vi "Experiment 7.VI"() -> ()   [LabVIEW 2017]
uses:
  <vilib>/DAQmx/write.llb/DAQmx Write (Analog DBL 1Chan 1Samp).vi
  <vilib>/DAQmx/write.llb/DAQmx Write (Digital 1D Bool NChan 1Samp 1Line).vi
  <vilib>/DAQmx/read.llb/DAQmx Read (Digital 1D Bool NChan 1Samp 1Line).vi
  <vilib>/DAQmx/read.llb/DAQmx Read (Analog 2D DBL NChan NSamp).vi
  <vilib>/DAQmx/create/channels.llb/DAQmx Create Channel (DI-Digital Input).vi
  <vilib>/DAQmx/create/channels.llb/DAQmx Create Channel (AI-Voltage-Basic).vi
  <vilib>/DAQmx/configure/timing.llb/DAQmx Timing (Sample Clock).vi
  <vilib>/DAQmx/create/channels.llb/DAQmx Create Channel (AO-Voltage-Basic).vi
  <vilib>/DAQmx/create/channels.llb/DAQmx Create Channel (DO-Digital Output).vi
  <vilib>/DAQmx/miscellaneous.llb/DAQmx Fill In Error Info.vi
panel:
  in  "Analogue Output":dbl(slide) scale=0.0..10.0
  out "Analogue Loopback":dbl[](graph)
  in  "Red LED":bool
  in  "Green LED":bool
  out "Button":bool
  out "Switch":bool
  in  "stop":bool
  out "Potentionmeter":dbl[](graph)
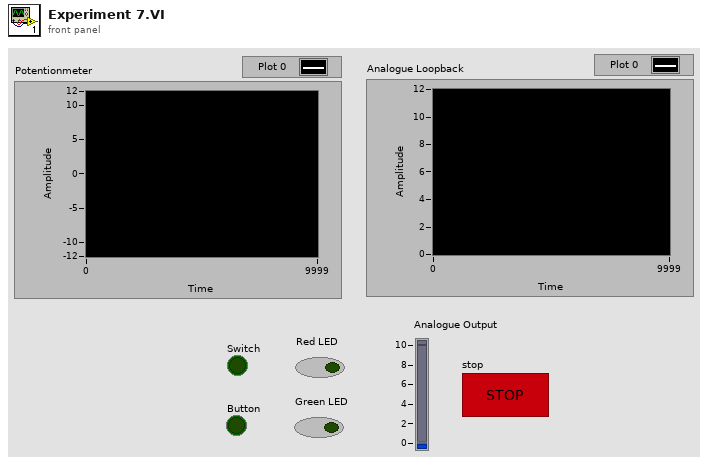
[diagram p1: front panel]
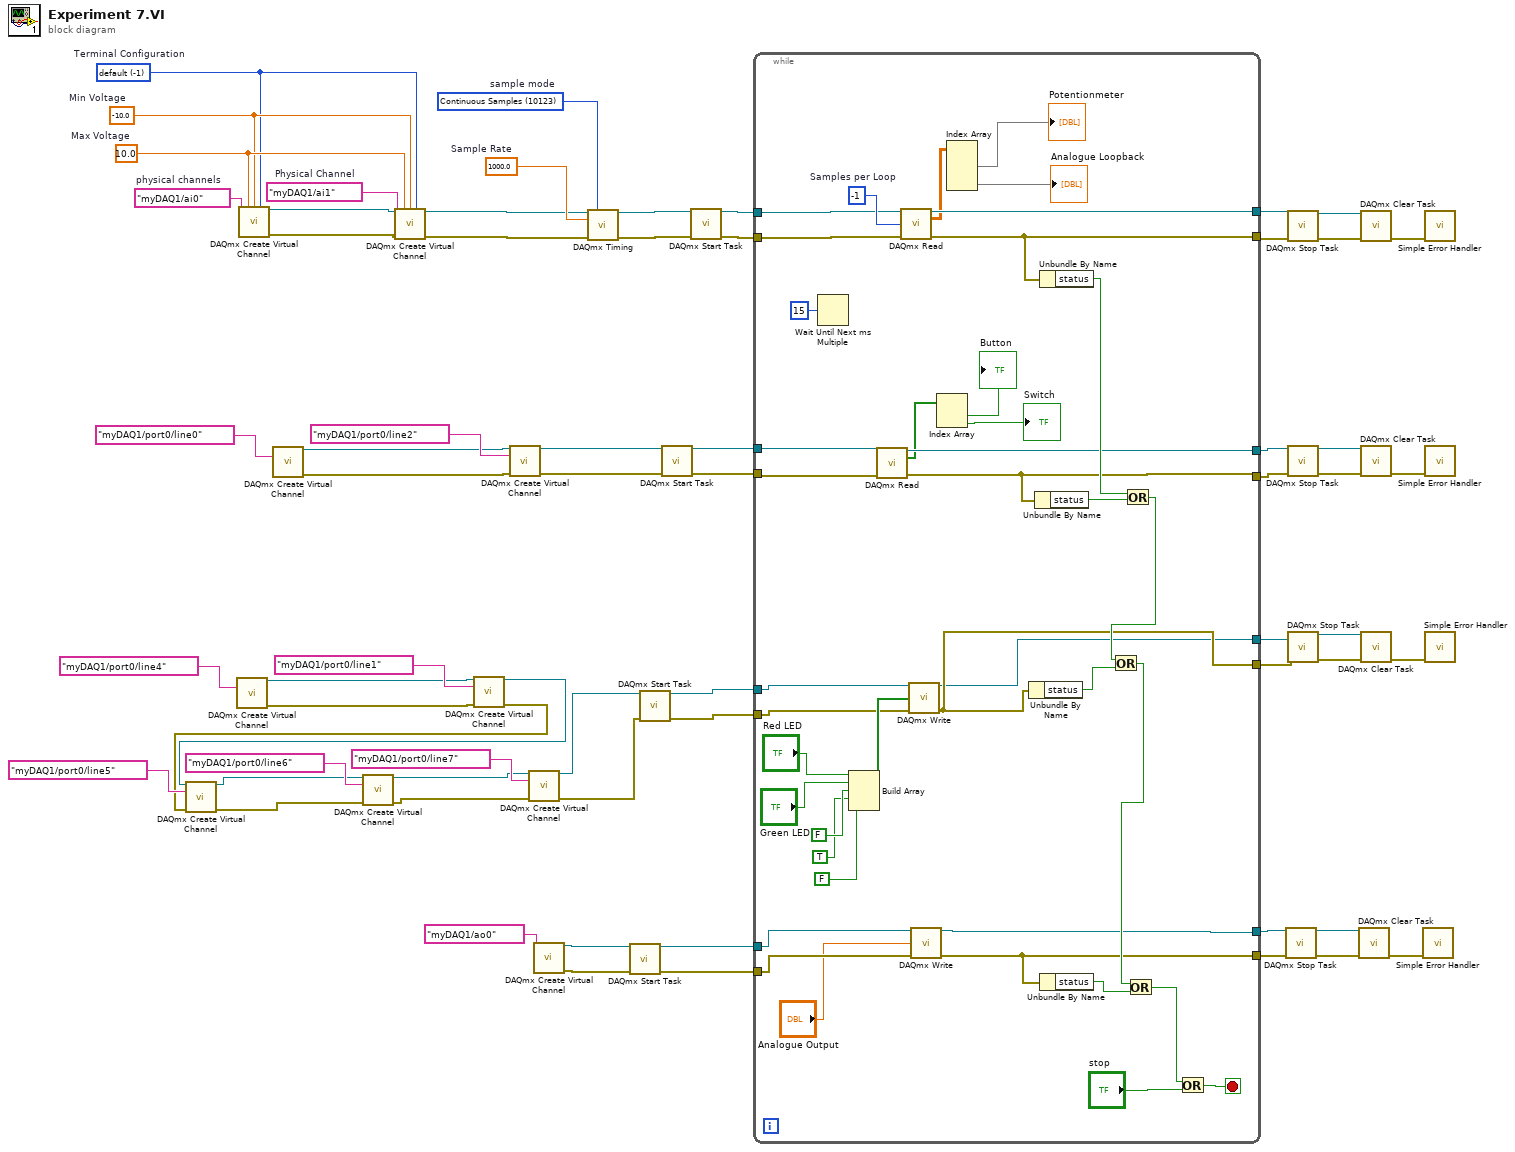
[diagram p0: block diagram]
diagram:
  w29 = tag "myDAQ1/ai0"  # physical channels
  w63 = 10123 items=["Finite Samples"=10178, "Continuous Samples"=10123, "Hardware Timed Single Point"=12522]  # sample mode
  w64 = 1000.0  # Sample Rate
  w26 = -1 items=["default"=-1, "RSE"=10083, "NRSE"=10078, "Differential"=10106, "Pseudodifferential"=12529]  # Terminal Configuration
  w27 = -10.0  # Min Voltage
  w28 = 10.0  # Max Voltage
  w65 = tag "myDAQ1/ai1"  # Physical Channel
  n1 = call-poly <vilib>:"DAQmx Create Virtual Channel.vi"("lines"=tag "myDAQ1/port0/line4") -> ("task out"=w16:refnum<k21>, "error out"=w15:errorcluster)  [unwired: 13 in]
  n2 = call-poly <vilib>:"DAQmx Create Virtual Channel.vi"("maximum value"=w28, "minimum value"=w27, "input terminal configuration"=w26, "physical channels"=w29) -> ("task out"=w30:refnum<k21>, "error out"=w31:errorcluster)  [unwired: 10 in]
  n3 = call-poly <vilib>:"DAQmx Create Virtual Channel.vi"("lines"=tag "myDAQ1/port0/line0") -> ("task out"=w41:refnum<k21>, "error out"=w40:errorcluster)  [unwired: 13 in]
  n4 = call-poly <vilib>:"DAQmx Create Virtual Channel.vi"("task in"=w30, "maximum value"=w28, "minimum value"=w27, "input terminal configuration"=w26, "physical channels"=w65, "error in"=w31) -> ("task out"=w61:refnum<k21>, "error out"=w62:errorcluster)  [unwired: 8 in]
  n5 = call-poly <vilib>:"DAQmx Create Virtual Channel.vi"("task in"=w16, "lines"=tag "myDAQ1/port0/line1", "error in"=w15) -> ("task out"=w10:refnum<k21>, "error out"=w5:errorcluster)  [unwired: 11 in]
  n6 = call-poly <vilib>:"DAQmx Create Virtual Channel.vi"("task in"=w10, "lines"=tag "myDAQ1/port0/line5", "error in"=w5) -> ("task out"=w9:refnum<k21>, "error out"=w6:errorcluster)  [unwired: 11 in]
  n7 = call-poly <vilib>:"DAQmx Create Virtual Channel.vi"("task in"=w9, "lines"=tag "myDAQ1/port0/line6", "error in"=w6) -> ("task out"=w8:refnum<k21>, "error out"=w7:errorcluster)  [unwired: 11 in]
  n8 = call-poly <vilib>:"DAQmx Create Virtual Channel.vi"("task in"=w41, "lines"=tag "myDAQ1/port0/line2", "error in"=w40) -> ("task out"=w50:refnum<k21>, "error out"=w49:errorcluster)  [unwired: 11 in]
  n9 = call-poly <vilib>:"DAQmx Create Virtual Channel.vi"("task in"=w8, "lines"=tag "myDAQ1/port0/line7", "error in"=w7) -> ("task out"=w4:refnum<k21>, "error out"=w3:errorcluster)  [unwired: 11 in]
  n10 = call-poly <vilib>:"DAQmx Create Virtual Channel.vi"("physical channels"=tag "myDAQ1/ao0") -> ("task out"=w22:refnum<k21>, "error out"=w21:errorcluster)  [unwired: 13 in]
  n11 = call-poly <vilib>:"DAQmx Timing.vi"("task/channels in"=w61, "sample mode"=w63, "rate"=w64, "error in"=w62) -> ("task out"=w60:refnum<k21>, "error out"=w59:errorcluster)  [unwired: 10 in]
  n12 = call <vilib>:"DAQmx Start Task.vi"("task/channels in"=w22, "error in"=w21) -> ("task out"=w19:refnum<k21>, "error out"=w18:errorcluster)  [unwired: 12 in]
  n13 = call <vilib>:"DAQmx Start Task.vi"("task/channels in"=w4, "error in"=w3) -> ("task out"=w33:refnum<k21>, "error out"=w32:errorcluster)  [unwired: 12 in]
  n14 = call <vilib>:"DAQmx Start Task.vi"("task/channels in"=w50, "error in"=w49) -> ("task out"=w48:refnum<k21>, "error out"=w47:errorcluster)  [unwired: 12 in]
  n15 = call <vilib>:"DAQmx Start Task.vi"("task/channels in"=w60, "error in"=w59) -> ("task out"=w58:refnum<k21>, "error out"=w57:errorcluster)  [unwired: 12 in]
  n16 = while {
    tunnel: w58 -> [w102]
    tunnel: w57 -> [w103]
    tunnel: [w99] -> w54
    tunnel: [w98] -> w53
    tunnel: w48 -> [w96]
    tunnel: w47 -> [w95]
    tunnel: [w94] -> w43
    tunnel: [w92] -> w42
    tunnel: [w86] -> w37
    tunnel: [w85] -> w38
    tunnel: w33 -> [w82]
    tunnel: w32 -> [w83]
    tunnel: w19 -> [w69]
    tunnel: w18 -> [w68]
    tunnel: [w70] -> w1
    tunnel: [w67] -> w2
    stop <- w101 stop-if-true
    w104 = -1  # Samples per Loop
    n17 = Wait Until Next ms Multiple(millisecond multiple=u32 15) -> ()  [unwired: 1 out]
    n18 = Build Array("Red LED", "Green LED", FALSE, TRUE, FALSE) -> (w84:bool[])
    n19 = call-poly <vilib>:"DAQmx Read.vi"("task/channels in"=w96, "error in"=w95) -> ("task out"=w92:refnum<k21>, "data"=w91:bool[], "error out"=w94:errorcluster)  [unwired: 11 in]
    n20 = call-poly <vilib>:"DAQmx Read.vi"("task/channels in"=w102, "number of samples per channel"=w104, "error in"=w103) -> ("task out"=w98:refnum<k21>, "data"=w78:dbl[][], "error out"=w99:errorcluster)  [unwired: 10 in]
    n21 = call-poly <vilib>:"DAQmx Write.vi"("task/channels in"=w82, "data"=w84, "error in"=w83) -> ("task out"=w85:refnum<k21>, "error out"=w86:errorcluster)  [unwired: 10 in, 1 out]
    n22 = call-poly <vilib>:"DAQmx Write.vi"("task/channels in"=w69, "data"="Analogue Output", "error in"=w68) -> ("task out"=w67:refnum<k21>, "error out"=w70:errorcluster)  [unwired: 10 in, 1 out]
    n23 = Index Array(array=w91) -> (element #1=→"Button":bool, element #2=→"Switch":bool)  [unwired: 2 in]
    n24 = Index Array(array=w78) -> (element #1=→"Potentionmeter":dbl[], element #2=→"Analogue Loopback":dbl[])  [unwired: 4 in]
    n25 = Unbundle By Name(w86) -> ("status"=w87:bool)
    n26 = Unbundle By Name(w94) -> ("status"=w93:bool)
    n27 = Unbundle By Name(w99) -> ("status"=w97:bool)
    n28 = Unbundle By Name(w70) -> ("status"=w76:bool)
    n29 = Or(x=w97, y=w93) -> (x .or. y?=w88:bool)
    n30 = Or(x=w88, y=w87) -> (x .or. y?=w74:bool)
    n31 = Or(x=w74, y=w76) -> (x .or. y?=w75:bool)
    n32 = Or(x=w75, y="stop") -> (x .or. y?=w101:bool)
  }
  n33 = call <vilib>:"DAQmx Stop Task.vi"("task/channels in"=w2, "error in"=w1) -> ("task out"=w25:refnum<k21>, "error out"=w24:errorcluster)  [unwired: 12 in]
  n34 = call <vilib>:"DAQmx Stop Task.vi"("task/channels in"=w53, "error in"=w54) -> ("task out"=w56:refnum<k21>, "error out"=w55:errorcluster)  [unwired: 12 in]
  n35 = call <vilib>:"DAQmx Stop Task.vi"("task/channels in"=w42, "error in"=w43) -> ("task out"=w46:refnum<k21>, "error out"=w45:errorcluster)  [unwired: 12 in]
  n36 = call <vilib>:"DAQmx Stop Task.vi"("task/channels in"=w38, "error in"=w37) -> ("task out"=w36:refnum<k21>, "error out"=w35:errorcluster)  [unwired: 12 in]
  n37 = call <vilib>:"DAQmx Clear Task.vi"("task in"=w25, "error in"=w24) -> ("error out"=w23:errorcluster)  [unwired: 13 in]
  n38 = call <vilib>:"DAQmx Clear Task.vi"("task in"=w56, "error in"=w55) -> ("error out"=w52:errorcluster)  [unwired: 13 in]
  n39 = call <vilib>:"DAQmx Clear Task.vi"("task in"=w46, "error in"=w45) -> ("error out"=w44:errorcluster)  [unwired: 13 in]
  n40 = call <vilib>:"DAQmx Clear Task.vi"("task in"=w36, "error in"=w35) -> ("error out"=w34:errorcluster)  [unwired: 13 in]
  n41 = call <vilib>:"Simple Error Handler.vi"("error in (no error)"=w23) -> ()  [unwired: 4 in, 5 out]
  n42 = call <vilib>:"Simple Error Handler.vi"("error in (no error)"=w52) -> ()  [unwired: 4 in, 5 out]
  n43 = call <vilib>:"Simple Error Handler.vi"("error in (no error)"=w44) -> ()  [unwired: 4 in, 5 out]
  n44 = call <vilib>:"Simple Error Handler.vi"("error in (no error)"=w34) -> ()  [unwired: 4 in, 5 out]
